vi "글로벌 3.vi"() -> ()   [LabVIEW 2014]
panel:
  out "문자열":string
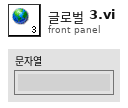
[diagram p1: front panel]
diagram:
